vi "Constructor.vi"(7 "ComparisonType":T1, 8 "error in":errorcluster, 9 "HigherBond":i64, 10 "LowerBound":i64, 11 "Name":string) -> (0 "error out":errorcluster, 3 "IntegerMeasureLimit":refnum<class "IntegerMeasureLimit.lvclass">)   [LabVIEW 2021, in "ProligentXMLGenerator.lvlib" / "IntegerMeasureLimit.lvclass"]
uses:
  IntegerMeasureLimit.lvclass
  IntegerMeasureLimit.lvclass/IntegerMeasureLimit.ctl
  MeasureLimit/MeasureLimit.lvclass
  Data.ctl
  Base/Integer/Integer.lvclass
  RangeMeasureLimit/RangeMeasureLimit.lvclass
  C:/Projects/proligent-xml-generator-labview/src/ProligentXMLGenerator/Measure/RangeMeasureLimit/RangeMeasureLimit.lvclass
  C:/Projects/proligent-xml-generator-labview/src/ProligentXMLGenerator/Measure/MeasureLimit/MeasureLimit.lvclass
  RangeMeasureLimit/ComparisonType.ctl
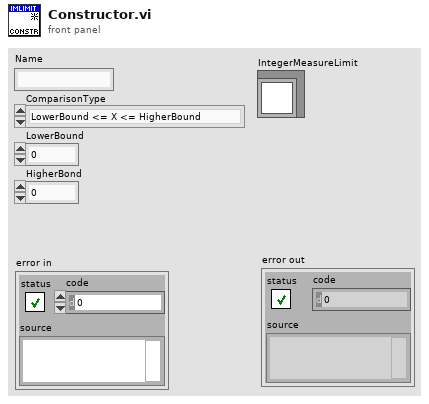
[diagram p1: front panel]
types:
  T1 = typedef "ProligentXMLGenerator.lvlib/RangeMeasureLimit.lvclass/ComparisonType.ctl" = enum16{"LowerBound <= X <= HigherBound", "LowerBound < X <= HigherBound", "LowerBound <= X < HigherBound", "LowerBound < X < HigherBound", "LowerBound <= X", "LowerBound < X", "X <= HigherBound", "X < HigherBound", "X == HigherBound", "X != HigherBound", "X <= LowerBound OR HigherBound <= X", "X < LowerBound OR HigherBound <= X", "X <= LowerBound OR HigherBound < X", "X < LowerBound OR HigherBound < X"}
  T2 = typedef "ProligentXMLGenerator.lvlib/IntegerMeasureLimit.lvclass/Data.ctl" = cluster{"LowerBound":refnum<class "Integer.lvclass">, "HigherBound":refnum<class "Integer.lvclass">}
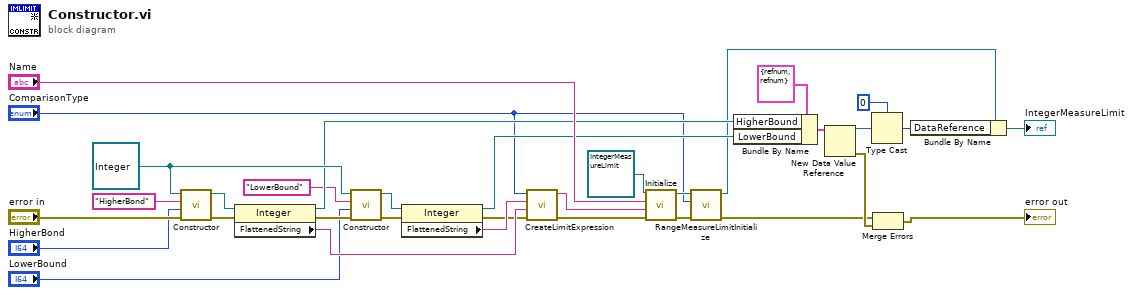
[diagram p0: block diagram]
diagram:
  w19 = refnum<class "Integer.lvclass"> refnum ("ProligentResultProcessor:Integer")
  n1 = call-dynamic "Constructor.vi"("error in"="error in", "Value"="HigherBond", "Name"="HigherBond", "Integer in"=w19) -> ("error out"=w20:errorcluster, "Integer out"=w15:refnum<class "Integer.lvclass">)  [unwired: 6 in]
  n2 = property class="Integer"(reference=w15, error in=w20) -> (reference out=w7:refnum<class "Integer.lvclass">, error out=w16:errorcluster, "FlattenedString"=w14:string)
  n3 = call-dynamic "Constructor.vi"("error in"=w16, "Value"="LowerBound", "Name"="LowerBound", "Integer in"=w19) -> ("error out"=w11:errorcluster, "Integer out"=w12:refnum<class "Integer.lvclass">)  [unwired: 6 in]
  n4 = property class="Integer"(reference=w12, error in=w11) -> (reference out=w8:refnum<class "Integer.lvclass">, error out=w9:errorcluster, "FlattenedString"=w10:string)
  n5 = call "CreateLimitExpression.vi"("error in"=w9, "HigherBound"=w14, "LowerBound"=w10, "ComparisonType"="ComparisonType") -> ("error out"=w24:errorcluster, "LimitExpression"=w23:string)  [unwired: 6 in]
  n6 = call "Initialize.vi"("error in"=w24, "LimitExpression"=w23, "Name"="Name", "MeasureLimit in"=refnum<class "IntegerMeasureLimit.lvclass"> refnum ("ProligentResultProcessor:RealMeasureLimit.lvclass")) -> ("error out"=w3:errorcluster, "MeasureLimit out"=w22:refnum<class "IntegerMeasureLimit.lvclass">)  [unwired: 6 in]
  n7 = call "RangeMeasureLimitInitialize.vi"("error in"=w3, "ComparisonType"="ComparisonType", "RangeMeasureLimit in"=w22) -> ("error out"=w2:errorcluster, "RangeMeasureLimit out"=w4:refnum<class "IntegerMeasureLimit.lvclass">)  [unwired: 7 in]
  n8 = Bundle By Name(cluster=T2 {"LowerBound"=refnum, "HigherBound"=refnum} ("Data"), "HigherBound"=w7, "LowerBound"=w8) -> (w29:T2)
  n9 = New Data Value Reference(data value=w29) -> (data value reference=w30:refnum<data-value>, error out=w33:errorcluster)  [unwired: 1 in]
  n10 = Type Cast(type=u64 0, x=w30) -> (*(type *) &x=w32:u64)
  n11 = Merge Errors(w2, w33) -> (→"error out":errorcluster)
  n12 = Bundle By Name(cluster=w4, "DataReference"=w32) -> (→"IntegerMeasureLimit":refnum<class "IntegerMeasureLimit.lvclass">)
